vi "Save_Cross_spectra_plots.vi"(0 "Plots to save":cluster{dbl, dbl, "2D data":dbl[]}[](array[cluster]) {"2D data" format="%.2f"; "?" format="%.2f"; "?" format="%.2f"}, 2 "Show Smooth":bool, 3 "U1":u16(ring), 4 "U2":u16(ring)) -> ()   [LabVIEW 2010]
uses:
  Globals/Meas_global.vi
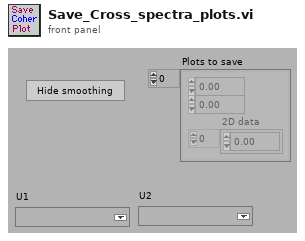
[diagram p1: front panel]
types:
  T1 = cluster{"Name":string, "X":dbl, "Y":dbl, "Z":dbl}[]
  T2 = cluster{"Name":string, "X":dbl, "Y":dbl, "Z":dbl}
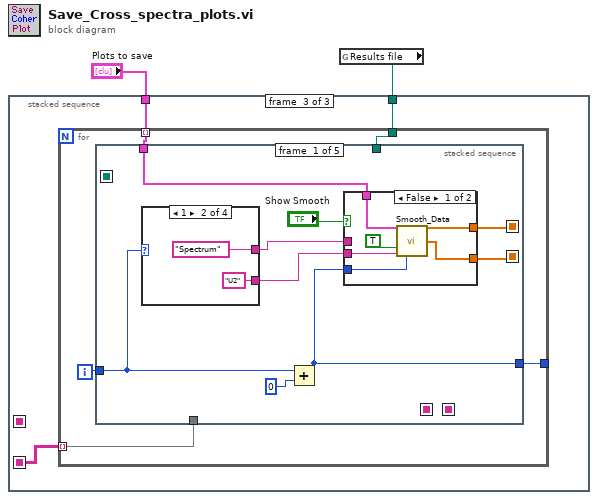
[diagram p0: block diagram]
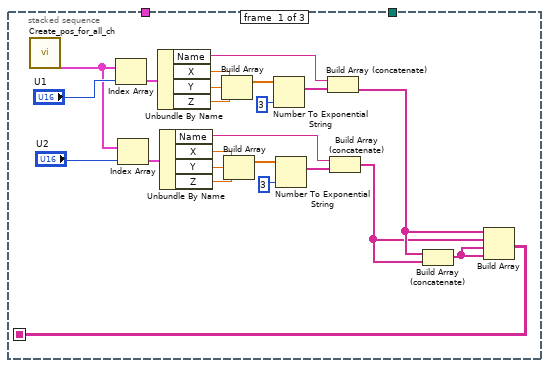
[diagram p2: hidden frame]
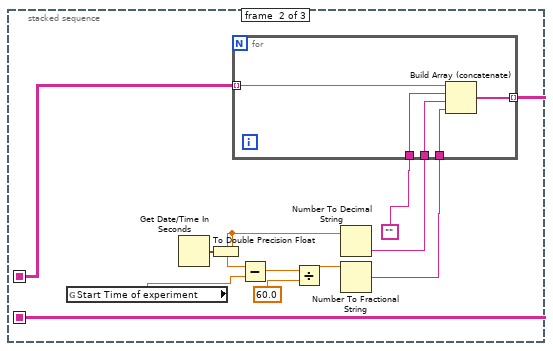
[diagram p3: hidden frame]
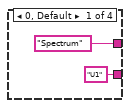
[diagram p4: hidden frame]
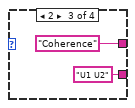
[diagram p5: hidden frame]
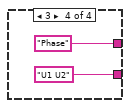
[diagram p6: hidden frame]
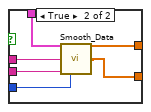
[diagram p7: hidden frame]
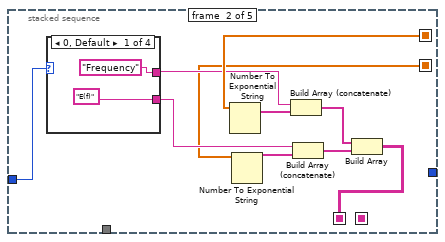
[diagram p8: hidden frame]
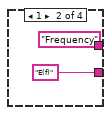
[diagram p9: hidden frame]
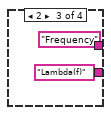
[diagram p10: hidden frame]
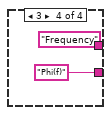
[diagram p11: hidden frame]
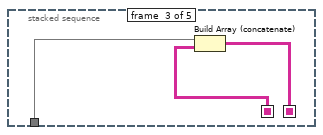
[diagram p12: hidden frame]
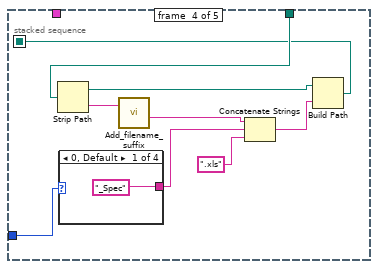
[diagram p13: hidden frame]
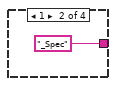
[diagram p14: hidden frame]
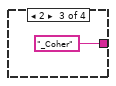
[diagram p15: hidden frame]
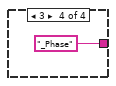
[diagram p16: hidden frame]
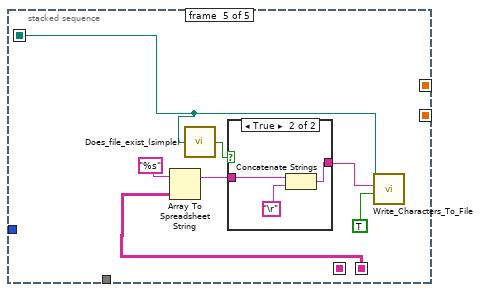
[diagram p17: hidden frame]
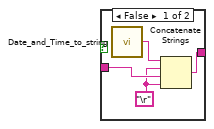
[diagram p18: hidden frame]
diagram:
  n1 = global read "Meas_global.vi" "Results file"() -> (w2:path)
  n2 = stacked-sequence {
    seq-local: [_ w36 _] -> [_ _ w44]
    seq-local: [w3 _ _] -> [_ w27 _]
    tunnel: w2 -> [_ _ w43]
    tunnel: "Plots to save" -> [_ _ w42]
    frame #0 {
      n3 = call "Create_pos_for_all_ch.vi"() -> ("Positions for all Ch"=w7:T1)  [unwired: 6 out]
      n4 = Index Array(array=w7, index="U1") -> (element=w20:T2)
      n5 = Index Array(array=w7, index="U2") -> (element=w15:T2)
      n6 = Unbundle By Name(w20) -> ("Name"=w18:string, "X"=w25:dbl, "Y"=w24:dbl, "Z"=w23:dbl)
      n7 = Unbundle By Name(w15) -> ("Name"=w17:string, "X"=w10:dbl, "Y"=w11:dbl, "Z"=w12:dbl)
      n8 = Build Array(w25, w24, w23) -> (w21:dbl[])
      n9 = Build Array(w10, w11, w12) -> (w14:dbl[])
      n10 = Number To Exponential String(number=w21, precision (6)=3) -> (E-format string=w19:string[])  [unwired: 2 out]
      n11 = Number To Exponential String(number=w14, precision (6)=3) -> (E-format string=w16:string[])  [unwired: 2 out]
      n12 = Build Array (concatenate)(w18, w19) -> (w6:string[])
      n13 = Build Array (concatenate)(w17, w16) -> (w5:string[])
      n14 = Build Array (concatenate)(w6, w5) -> (w4:string[])
      n15 = Build Array(w6, w5, w4, w4) -> (w3:string[][])
    }
    frame #1 {
      n16 = global read "Meas_global.vi" "Start Time of experiment"() -> (w29:dbl)
      n17 = Get Date/Time In Seconds() -> (seconds since 1Jan1904=w26:timestamp)
      n18 = To Double Precision Float(number=w26) -> (double precision float=w28:dbl)
      n19 = Subtract(x=w28, y=w29) -> (x-y=w34:dbl)
      n20 = Divide(x=w34, y=60.0) -> (x/y=w33:dbl)
      n21 = Number To Decimal String(number=w28) -> (decimal integer string=w32:string)  [unwired: 1 out]
      n22 = Number To Fractional String(number=w33) -> (F-format string=w31:string)  [unwired: 3 out]
      n23 = for {
        tunnel: [w41] -> w36 mode=indexing
        tunnel: w32 -> [w40]
        tunnel: w31 -> [w39]
        tunnel: "" -> [w38]
        tunnel: w27 -> [w37] mode=indexing
        n24 = Build Array (concatenate)(w37, w38, w40, w39) -> (w41:string[])
      }
    }
    frame #2 {
      n25 = for {
        tunnel: w42 -> [w49] mode=indexing
        tunnel: [w47] -> _
        tunnel: w44 -> [w46] mode=indexing
        tunnel: w43 -> [w45]
        i -> [w48]
        n26 = stacked-sequence {
          seq-local: [_ _ w98 _ _] -> [_ _ _ _ w115]
          seq-local: [w56 _ _ _ _] -> [_ w84 _ _ _]
          seq-local: [w55 _ _ _ _] -> [_ w81 _ _ _]
          seq-local: [_ w80 _ _ _] -> [_ _ w99 _ _]
          seq-local: [_ _ _ w102 _] -> [_ _ _ _ w113]
          tunnel: w49 -> [w58 _ _ _ _]
          tunnel: w48 -> [w53 w79 _ w101 _]
          tunnel: [w57 _ _ _ _] -> w47
          tunnel: w45 -> [_ _ _ w103 _]
          tunnel: w46 -> [_ _ w97 _ _]
          frame #0 {
            n27 = case shown="1" w53 {
              tunnel: ["Spectrum" "Spectrum" "Coherence" "Phase"] -> w52
              tunnel: ["U1" "U2" "U1 U2" "U1 U2"] -> w51
              frame 0, Default {
              }
              frame 1 {
              }
              frame 2 {
              }
              frame 3 {
              }
            }
            n28 = Add(x=w53, y=0) -> (x+y=w57:i32)
            n29 = case shown="False" "Show Smooth" {
              tunnel: w58 -> [w72 w78]
              tunnel: w57 -> [w70 w77]
              tunnel: w51 -> [w69 w76]
              tunnel: [w68 w75] -> w56
              tunnel: [w67 w74] -> w55
              tunnel: w52 -> [_ w73]
              frame False {
                n30 = call "Smooth_Data.vi"("Plot cluster"=w72, "OK"=TRUE, "Trace name"=w69, "Trace No"=w70) -> ("X array Out"=w68:dbl[], "Y array Out"=w67:dbl[])  [unwired: 2 in, 8 out]
              }
              frame True {
                n31 = call "Smooth_Data.vi"("Plot cluster"=w78, "Plot type"=w73, "Trace name"=w76, "Trace No"=w77) -> ("X array Out"=w75:dbl[], "Y array Out"=w74:dbl[])  [unwired: 2 in, 8 out]
              }
            }
          }
          frame #1 {
            n32 = case shown="0, Default" w79 {
              tunnel: ["Frequency" "Frequency" "Frequency" "Frequency"] -> w83
              tunnel: ["E(f)" "E(f)" "Lambda(f)" "Phi(f)"] -> w82
              frame 0, Default {
              }
              frame 1 {
              }
              frame 2 {
              }
              frame 3 {
              }
            }
            n33 = Number To Exponential String(number=w84) -> (E-format string=w87:string[])  [unwired: 3 out]
            n34 = Number To Exponential String(number=w81) -> (E-format string=w88:string[])  [unwired: 3 out]
            n35 = Build Array (concatenate)(w83, w87) -> (w85:string[])
            n36 = Build Array (concatenate)(w82, w88) -> (w86:string[])
            n37 = Build Array(w85, w86) -> (w80:string[][])
          }
          frame #2 {
            n38 = Build Array (concatenate)(w97, w99) -> (w98:string[][])
          }
          frame #3 {
            n39 = Strip Path(path=w103) -> (stripped path=w108:path, name=w104:string)
            n40 = case shown="0, Default" w101 {
              tunnel: ["_Spec" "_Spec" "_Coher" "_Phase"] -> w100
              frame 0, Default {
              }
              frame 1 {
              }
              frame 2 {
              }
              frame 3 {
              }
            }
            n41 = call "Add_filename_suffix.vi"("Filename"=w104) -> ("Base name"=w105:string)  [unwired: 1 in, 3 out]
            n42 = Concatenate Strings(w105, w100, ".xls" ("string")) -> (w107:string)
            n43 = Build Path(base path=w108, name or relative path=w107) -> (appended path=w102:path)
          }
          frame #4 {
            n44 = Array To Spreadsheet String(array=w115, 3:"%s") -> (spreadsheet string=w116:string)  [unwired: 1 out]
            n45 = call "Does_file_exist_(simple).vi"("Pathname"=w113) -> ("exists?"=w114:bool)
            n46 = case shown="True" w114 {
              tunnel: w116 -> [w123 w126]
              tunnel: [w121 w125] -> w117
              frame False {
                w122 = "\r"
                n47 = call "Date_and_Time_to_string.vi"() -> ("Date and time (spreadsheet)"=w120:string)
                n48 = Concatenate Strings(w120, w122, w123, w122) -> (w121:string)
              }
              frame True {
                n49 = Concatenate Strings(w126, "\r") -> (w125:string)
              }
            }
            n50 = call "Write_Characters_To_File.vi"("file path (dialog if empty)"=w113, "character string"=w117, "append to file? (new file:F)"=TRUE) -> ()  [unwired: 2 in, 4 out]
          }
        }
      }
    }
  }
